vi "Load.vi"(8 "error in":errorcluster, 10 "Source":string, 11 "Config From JSON in":refnum<class "Config from JSON.lvclass">) -> (0 "error out":errorcluster, 3 "Config From JSON out":refnum<class "Config from JSON.lvclass">)   [LabVIEW 2024, in "Config from JSON.lvclass"]
uses:
  Config from JSON.lvclass
  Config from JSON.lvclass/Config from JSON.ctl
  <vilib>/JDP Science/JSONtext/Config Files/Config File.lvclass
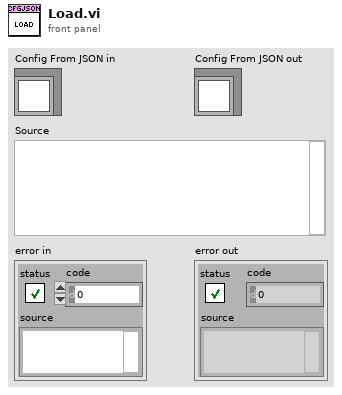
[diagram p1: front panel]
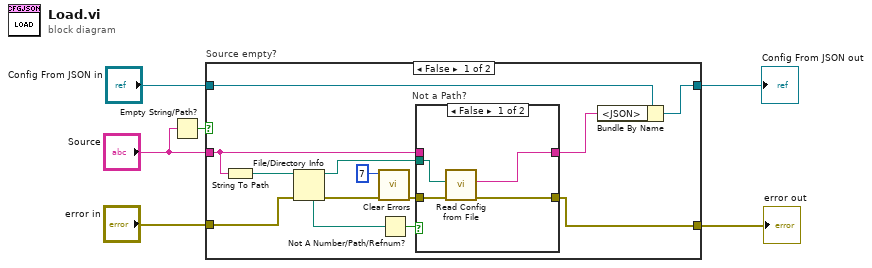
[diagram p0: block diagram]
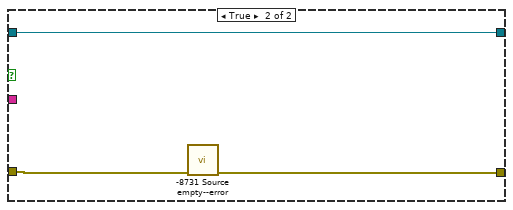
[diagram p3: hidden frame]
diagram:
  n1 = Empty String/Path?(string/path="Source") -> (empty?=w2:bool)
  n2 = case "Source empty?" shown="False" w2 {
    tunnel: "Config From JSON in" -> [w19 w27]
    tunnel: [w18 w26] -> w5
    tunnel: [w17 w27] -> w4
    tunnel: "Source" -> [w15 _]
    tunnel: "error in" -> [w9 w28]
    frame False {
      n3 = String To Path(string=w15) -> (path=w14:path)
      n4 = File/Directory Info(path=w14, error in=w9) -> (path out=w13:path, error out=w10:errorcluster, resolved path=w12:path)  [unwired: 4 out]
      n5 = call <vilib>:"Clear Errors.vi"("error in (no error)"=w10, "specific error code to clear (0: all)"=7) -> ("error out"=w8:errorcluster)  [unwired: 4 in, 1 out]
      n6 = Not A Number/Path/Refnum?(number/path/refnum=w12) -> (NaN/Path/Refnum?=w11:bool)
      n7 = case "Not a Path?" shown="False" w11 {
        tunnel: [w23 w25] -> w18
        tunnel: [w20 w24] -> w16
        tunnel: w8 -> [w22 w25]
        tunnel: w13 -> [w21 _]
        tunnel: w15 -> [_ w24]
        frame False {
          n8 = call <vilib>:"Read Config from File.vi"("error in (no error)"=w22, "config file path"=w21) -> ("error out"=w23:errorcluster, "<JSON>Config"=w20:string)  [unwired: 6 in, 2 out]
        }
        frame True {
        }
      }
      n9 = Bundle By Name(cluster=w19, "<JSON>"=w16) -> (w17:refnum<class "Config from JSON.lvclass">)
    }
    frame True {
      n10 = call "-8731 Source empty--error.vi"("error in"=w28) -> ("error out"=w26:errorcluster)  [unwired: 10 in]
    }
  }
  "error out" <- w5
  "Config From JSON out" <- w4
